vi "nxn.vi"() -> ()   [LabVIEW 2024]
panel:
  out "out":dbl[][](array[numeric])
  in  "n":i32
  in  "in":dbl[](array[numeric])
  # "out n x n"
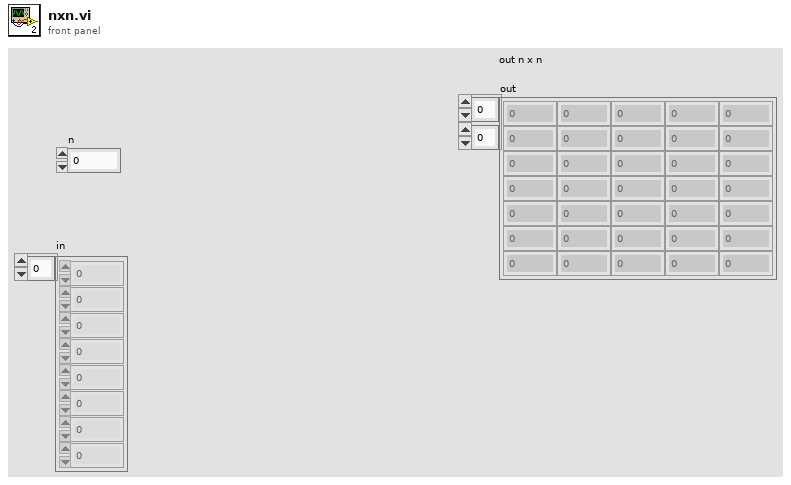
[diagram p1: front panel]
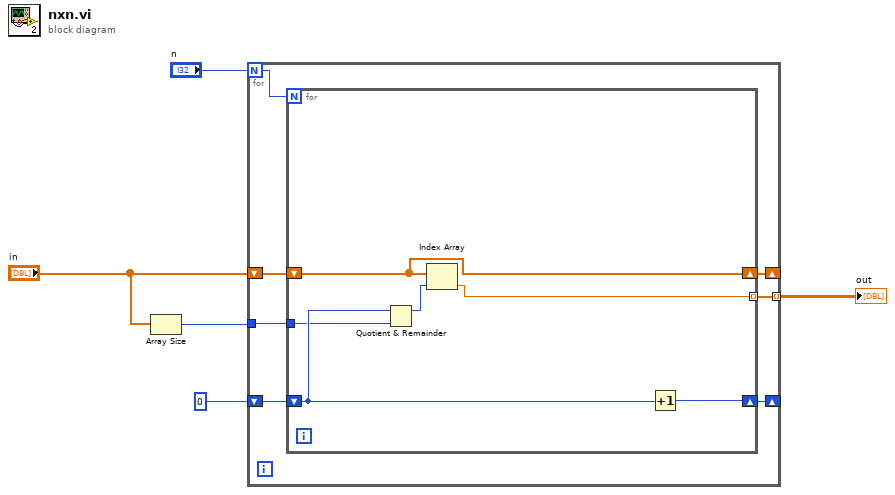
[diagram p0: block diagram]
diagram:
  n1 = Array Size(array="in") -> (size(s)=w3:i32)
  n2 = for {
    N: "n" -> [w6]
    shift-right: [w11] -> _
    shift-left: "in" -> [w12]
    tunnel: w3 -> [w10]
    shift-right: [w8] -> _
    shift-left: 0 -> [w9]
    tunnel: [w7] -> w1 mode=indexing
    n3 = for {
      N: w6 -> [_]
      shift-right: [w13] -> w11
      shift-left: w12 -> [w13]
      tunnel: w10 -> [w14]
      shift-right: [w17] -> w8
      shift-left: w9 -> [w18]
      tunnel: [w15] -> w7 mode=indexing
      n4 = Quotient & Remainder(x=w18, y=w14) -> (x-y*floor(x/y)=w16:i32)  [unwired: 1 out]
      n5 = Index Array(array=w13, index=w16) -> (element=w15:dbl)
      n6 = Increment(x=w18) -> (x+1=w17:i32)
    }
  }
  "out" <- w1
